vi "Read Actuator Settings.vi"(8 "error in (no error)":errorcluster, 11 "Boot Loader in":refnum<class "Boot Loader.lvclass">) -> (0 "error out":errorcluster, 2 "HPSettings":T1, 3 "Boot Loader out":refnum<class "Boot Loader.lvclass">)   [LabVIEW 2016, in "Boot Loader.lvclass"]
uses:
  Boot Loader.lvclass
  common_rt_hpilc/DataTypes/HPSettings.ctl
  common_rt_ilc/DataTypes/ILCSettings.ctl
  Settings/Settings.lvclass
  common_rt_ilc/RTILC.lvlib
  common_rt_hpilc/RTHPILC.lvlib
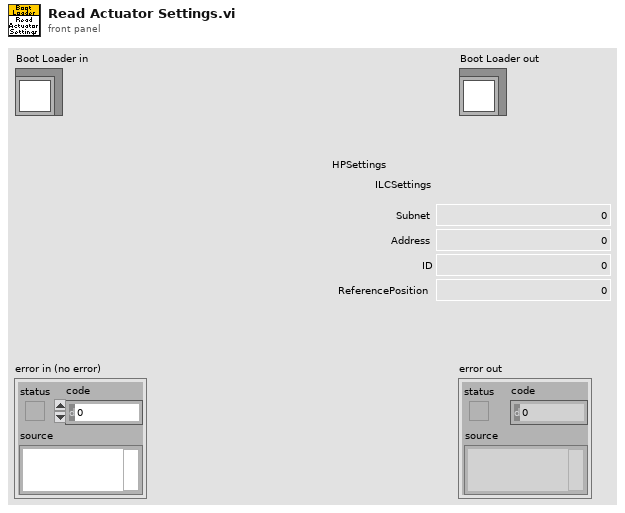
[diagram p1: front panel]
types:
  T1 = typedef "RTHPILC.lvlib/HPSettings.ctl" = cluster{"ILCSettings":T2, "ID":i16, "ReferencePosition":i32}
  T2 = typedef "RTILC.lvlib/ILCSettings.ctl" = cluster{"Subnet":u8, "Address":u8}
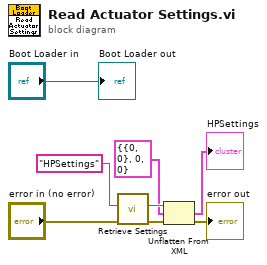
[diagram p0: block diagram]
diagram:
  n1 = call "Retrieve Settings.vi"("error in (no error)"="error in (no error)", "configName"="HPSettings") -> ("error out"=w4:errorcluster, "xmlConfig"=w7:string)  [unwired: 7 in, 1 out]
  n2 = Unflatten From XML(xml string=w7, type=T1 {"ILCSettings"={"Subnet"=0, "Address"=0}, "ID"=0, "ReferencePosition"=0} ("FASettings"), error in (no error)=w4) -> (value=→"HPSettings":T1, error out=→"error out":errorcluster)
  "Boot Loader out" <- "Boot Loader in"
